vi "Threshold Alert.vi"(8 "error in (no error)":errorcluster, 11 "Threshold Alert Data":T2) -> (0 "error out":errorcluster)   [LabVIEW 2018]
doc: "This subVI enqueues the named action in to the communications queue along with the input data."
uses:
  Private Controls/Module Action.ctl
  Testing UI 2.lvlib
  Private Controls/Module Data.ctl
  Top Level/Shared Controls/Threshold Alert Data.ctl
panel:
  in  "Action":T1=enum."Threshold ALERT"
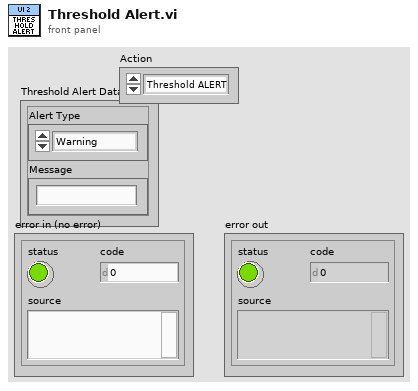
[diagram p1: front panel]
types:
  T1 = typedef "Testing UI 2.lvlib/Module Action.ctl" = enum8{"Init", "Error", "Exit", "Send Control Vals", "Update Indicators", "Load APU Setup", "Update APU Name", "Threshold ALERT", "Update Borders", "Update Test Information"}
  T2 = typedef "Threshold Alert Data.ctl" = cluster{"Alert Type":enum32{"Warning", "NormShutdown", "E-Stop"}, "Message":string}
  T3 = typedef "Testing UI 2.lvlib/Module Data.ctl" = cluster{"Data":variant, "Action":T4}
  T4 = typedef "Testing UI 2.lvlib/Module Action.ctl" = enum8{"Init", "Error", "Exit", "Timeout", "Load APU Setup", "Update Borders", "Update Test Information"}
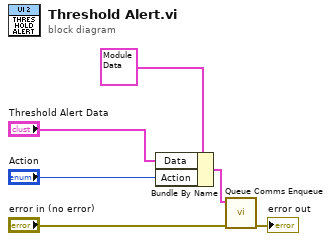
[diagram p0: block diagram]
diagram:
  n1 = Bundle By Name(cluster=T3 {"Data"=variant, "Action"=enum."Init"} ("element"), "Data"="Threshold Alert Data", "Action"="Action") -> (w5:T3)
  n2 = call "Queue Comms Enqueue.vi"("error in (no error)"="error in (no error)", "element"=w5) -> ("error out"=→"error out":errorcluster)  [unwired: 9 in]
